vi "Eye Movement Analyser.vi"(7 "Data Output":T12) -> ()   [LabVIEW 2016] (continued)
                  w628 = T14[] [] items=["--- System ---", "Panel Monitoring", "Check Save Status", "Initialize", "Initialise GUI", "Quit", "--- Import ---", "Desaccade Time Data", "Desaccade Time Data Background", "Paint Delete", "Load Batch Log File", "Make Batch List", "Update Batch List", "Delete Batch List", "Delete Temporary LVS", "Save Temporary LVS", "Check for Batch LVS", "Process 3D Chinchilla", "Find default parameter", "Mars3D old", "Chair", "EyeSeeCam", "Open last session", "Save RAW", "Auto Impulse Parameter", "Save Image", "Wireless", "Process Coils Data", "Process JHOC Data", "Process Animal Data", "Australian Data", "ASCII", "Mars 3D", "Mars 3D Training", "Position Mean Plugin", "plot generator plugin", "Human VOG system", "Optotrak", "spline", "COR", "galvanic", "Generate New Time Plot", "Make off and gains permanent", "Generate New Impulse Plot", "Defer Impulse Plot", "Fill Impulse Plot Data", "Scale Impulse Plot", "Un-Defer Impulse Plot", "Snap Impulse Cursor", "Extract Saccades", "Impulse Analyser", "NTA", "Acceleration", "Saccade Velocity", "Horizontal Align", "Vertical Align", "Delete Impulse", "Cut Before", "Cut After", "Filter Data", "Undo Last", "Redo", "Mean and STD", "Group Analyser", "Generate Report", "Phase Plots", "Gain and Phase", "Example Plugin", "Time Constant Plugin", "Export Data", "Export Time Series Data", "Append Data", "Save Data", "Load Data", "Cut in Range", "Keep in range", "Stop"] ("State stack IN")
                  n341 = event-data() -> ()  [unwired: 1 in, 2 out]
                }
                event "Time Constant Plugin": Mouse Down {
                  w631 = T14[] [enum."Time Constant Plugin"] items=["--- System ---", "Panel Monitoring", "Check Save Status", "Initialize", "Initialise GUI", "Quit", "--- Import ---", "Desaccade Time Data", "Desaccade Time Data Background", "Paint Delete", "Load Batch Log File", "Make Batch List", "Update Batch List", "Delete Batch List", "Delete Temporary LVS", "Save Temporary LVS", "Check for Batch LVS", "Process 3D Chinchilla", "Find default parameter", "Mars3D old", "Chair", "EyeSeeCam", "Open last session", "Save RAW", "Auto Impulse Parameter", "Save Image", "Wireless", "Process Coils Data", "Process JHOC Data", "Process Animal Data", "Australian Data", "ASCII", "Mars 3D", "Mars 3D Training", "Position Mean Plugin", "plot generator plugin", "Human VOG system", "Optotrak", "spline", "COR", "galvanic", "Generate New Time Plot", "Make off and gains permanent", "Generate New Impulse Plot", "Defer Impulse Plot", "Fill Impulse Plot Data", "Scale Impulse Plot", "Un-Defer Impulse Plot", "Snap Impulse Cursor", "Extract Saccades", "Impulse Analyser", "NTA", "Acceleration", "Saccade Velocity", "Horizontal Align", "Vertical Align", "Delete Impulse", "Cut Before", "Cut After", "Filter Data", "Undo Last", "Redo", "Mean and STD", "Group Analyser", "Generate Report", "Phase Plots", "Gain and Phase", "Example Plugin", "Time Constant Plugin", "Export Data", "Export Time Series Data", "Append Data", "Save Data", "Load Data", "Cut in Range", "Keep in range", "Stop"] ("State stack IN")
                  n342 = event-data() -> ()  [unwired: 1 in, 8 out]
                }
                event "Main Sequence Saccade": Mouse Down {
                  w634 = T14[] [enum."Extract Saccades"] items=["--- System ---", "Panel Monitoring", "Check Save Status", "Initialize", "Initialise GUI", "Quit", "--- Import ---", "Desaccade Time Data", "Desaccade Time Data Background", "Paint Delete", "Load Batch Log File", "Make Batch List", "Update Batch List", "Delete Batch List", "Delete Temporary LVS", "Save Temporary LVS", "Check for Batch LVS", "Process 3D Chinchilla", "Find default parameter", "Mars3D old", "Chair", "EyeSeeCam", "Open last session", "Save RAW", "Auto Impulse Parameter", "Save Image", "Wireless", "Process Coils Data", "Process JHOC Data", "Process Animal Data", "Australian Data", "ASCII", "Mars 3D", "Mars 3D Training", "Position Mean Plugin", "plot generator plugin", "Human VOG system", "Optotrak", "spline", "COR", "galvanic", "Generate New Time Plot", "Make off and gains permanent", "Generate New Impulse Plot", "Defer Impulse Plot", "Fill Impulse Plot Data", "Scale Impulse Plot", "Un-Defer Impulse Plot", "Snap Impulse Cursor", "Extract Saccades", "Impulse Analyser", "NTA", "Acceleration", "Saccade Velocity", "Horizontal Align", "Vertical Align", "Delete Impulse", "Cut Before", "Cut After", "Filter Data", "Undo Last", "Redo", "Mean and STD", "Group Analyser", "Generate Report", "Phase Plots", "Gain and Phase", "Example Plugin", "Time Constant Plugin", "Export Data", "Export Time Series Data", "Append Data", "Save Data", "Load Data", "Cut in Range", "Keep in range", "Stop"] ("State stack IN")
                  n343 = event-data() -> ()  [unwired: 1 in, 8 out]
                }
                event Menu Selection (User) {
                  n344 = event-data() -> ("ItemTag"=w640:string)  [unwired: 1 in, 6 out]
                  n345 = case shown="\"About\"" w640 {
                    tunnel: [w641 w642 _ w643 w644] -> w637
                    frame "False", Default {
                      w641 = T14[] [enum."Panel Monitoring"] items=["--- System ---", "Panel Monitoring", "Check Save Status", "Initialize", "Initialise GUI", "Quit", "--- Import ---", "Desaccade Time Data", "Desaccade Time Data Background", "Paint Delete", "Load Batch Log File", "Make Batch List", "Update Batch List", "Delete Batch List", "Delete Temporary LVS", "Save Temporary LVS", "Check for Batch LVS", "Process 3D Chinchilla", "Find default parameter", "Mars3D old", "Chair", "EyeSeeCam", "Open last session", "Save RAW", "Auto Impulse Parameter", "Save Image", "Wireless", "Process Coils Data", "Process JHOC Data", "Process Animal Data", "Australian Data", "ASCII", "Mars 3D", "Mars 3D Training", "Position Mean Plugin", "plot generator plugin", "Human VOG system", "Optotrak", "spline", "COR", "galvanic", "Generate New Time Plot", "Make off and gains permanent", "Generate New Impulse Plot", "Defer Impulse Plot", "Fill Impulse Plot Data", "Scale Impulse Plot", "Un-Defer Impulse Plot", "Snap Impulse Cursor", "Extract Saccades", "Impulse Analyser", "NTA", "Acceleration", "Saccade Velocity", "Horizontal Align", "Vertical Align", "Delete Impulse", "Cut Before", "Cut After", "Filter Data", "Undo Last", "Redo", "Mean and STD", "Group Analyser", "Generate Report", "Phase Plots", "Gain and Phase", "Example Plugin", "Time Constant Plugin", "Export Data", "Export Time Series Data", "Append Data", "Save Data", "Load Data", "Cut in Range", "Keep in range", "Stop"]  # State Stack (out)
                    }
                    frame "Load Batch-Log File" {
                      w642 = T14[] [enum."Load Batch Log File"] items=["--- System ---", "Panel Monitoring", "Check Save Status", "Initialize", "Initialise GUI", "Quit", "--- Import ---", "Desaccade Time Data", "Desaccade Time Data Background", "Paint Delete", "Load Batch Log File", "Make Batch List", "Update Batch List", "Delete Batch List", "Delete Temporary LVS", "Save Temporary LVS", "Check for Batch LVS", "Process 3D Chinchilla", "Find default parameter", "Mars3D old", "Chair", "EyeSeeCam", "Open last session", "Save RAW", "Auto Impulse Parameter", "Save Image", "Wireless", "Process Coils Data", "Process JHOC Data", "Process Animal Data", "Australian Data", "ASCII", "Mars 3D", "Mars 3D Training", "Position Mean Plugin", "plot generator plugin", "Human VOG system", "Optotrak", "spline", "COR", "galvanic", "Generate New Time Plot", "Make off and gains permanent", "Generate New Impulse Plot", "Defer Impulse Plot", "Fill Impulse Plot Data", "Scale Impulse Plot", "Un-Defer Impulse Plot", "Snap Impulse Cursor", "Extract Saccades", "Impulse Analyser", "NTA", "Acceleration", "Saccade Velocity", "Horizontal Align", "Vertical Align", "Delete Impulse", "Cut Before", "Cut After", "Filter Data", "Undo Last", "Redo", "Mean and STD", "Group Analyser", "Generate Report", "Phase Plots", "Gain and Phase", "Example Plugin", "Time Constant Plugin", "Export Data", "Export Time Series Data", "Append Data", "Save Data", "Load Data", "Cut in Range", "Keep in range", "Stop"]  # State Stack (out)
                    }
                    frame "About" {
                      n346 = call "About.vi"() -> ()  [unwired: 12 in]
                    }
                    frame "Open" {
                      w643 = T14[] [enum."Load Data"] items=["--- System ---", "Panel Monitoring", "Check Save Status", "Initialize", "Initialise GUI", "Quit", "--- Import ---", "Desaccade Time Data", "Desaccade Time Data Background", "Paint Delete", "Load Batch Log File", "Make Batch List", "Update Batch List", "Delete Batch List", "Delete Temporary LVS", "Save Temporary LVS", "Check for Batch LVS", "Process 3D Chinchilla", "Find default parameter", "Mars3D old", "Chair", "EyeSeeCam", "Open last session", "Save RAW", "Auto Impulse Parameter", "Save Image", "Wireless", "Process Coils Data", "Process JHOC Data", "Process Animal Data", "Australian Data", "ASCII", "Mars 3D", "Mars 3D Training", "Position Mean Plugin", "plot generator plugin", "Human VOG system", "Optotrak", "spline", "COR", "galvanic", "Generate New Time Plot", "Make off and gains permanent", "Generate New Impulse Plot", "Defer Impulse Plot", "Fill Impulse Plot Data", "Scale Impulse Plot", "Un-Defer Impulse Plot", "Snap Impulse Cursor", "Extract Saccades", "Impulse Analyser", "NTA", "Acceleration", "Saccade Velocity", "Horizontal Align", "Vertical Align", "Delete Impulse", "Cut Before", "Cut After", "Filter Data", "Undo Last", "Redo", "Mean and STD", "Group Analyser", "Generate Report", "Phase Plots", "Gain and Phase", "Example Plugin", "Time Constant Plugin", "Export Data", "Export Time Series Data", "Append Data", "Save Data", "Load Data", "Cut in Range", "Keep in range", "Stop"] ("State Stack (out)")
                    }
                    frame "Quit" {
                      w644 = T14[] [enum."Quit"] items=["--- System ---", "Panel Monitoring", "Check Save Status", "Initialize", "Initialise GUI", "Quit", "--- Import ---", "Desaccade Time Data", "Desaccade Time Data Background", "Paint Delete", "Load Batch Log File", "Make Batch List", "Update Batch List", "Delete Batch List", "Delete Temporary LVS", "Save Temporary LVS", "Check for Batch LVS", "Process 3D Chinchilla", "Find default parameter", "Mars3D old", "Chair", "EyeSeeCam", "Open last session", "Save RAW", "Auto Impulse Parameter", "Save Image", "Wireless", "Process Coils Data", "Process JHOC Data", "Process Animal Data", "Australian Data", "ASCII", "Mars 3D", "Mars 3D Training", "Position Mean Plugin", "plot generator plugin", "Human VOG system", "Optotrak", "spline", "COR", "galvanic", "Generate New Time Plot", "Make off and gains permanent", "Generate New Impulse Plot", "Defer Impulse Plot", "Fill Impulse Plot Data", "Scale Impulse Plot", "Un-Defer Impulse Plot", "Snap Impulse Cursor", "Extract Saccades", "Impulse Analyser", "NTA", "Acceleration", "Saccade Velocity", "Horizontal Align", "Vertical Align", "Delete Impulse", "Cut Before", "Cut After", "Filter Data", "Undo Last", "Redo", "Mean and STD", "Group Analyser", "Generate Report", "Phase Plots", "Gain and Phase", "Example Plugin", "Time Constant Plugin", "Export Data", "Export Time Series Data", "Append Data", "Save Data", "Load Data", "Cut in Range", "Keep in range", "Stop"] ("State Stack (out)")
                    }
                  }
                }
                event "Asymmetry Plot": Mouse Up {
                  n347 = event-data() -> ()  [unwired: 1 in, 8 out]
                  n348 = Unbundle By Name(w651) -> ("No. Imp"=w645:i32)
                  n349 = property on="Impulse Trace" class="WFGraph (strict)"() -> ("Value"=w653:cluster{dbl, dbl, "Impulses":dbl[][]})  [unwired: 2 in, 2 out]
                  n350 = Unbundle By Name(w653) -> ("Impulses"=w650:dbl[][])
                  n351 = Array Subset(array=w650, index (row)=0 ("index"), length (row)=w645) -> (w649:dbl[][])  [unwired: 2 in]
                  n352 = Array Subset(array=w650, index (row)=w645) -> (w648:dbl[][])  [unwired: 3 in]
                  n353 = for {
                    tunnel: w649 -> [w656] mode=indexing
                    tunnel: w648 -> [w655] mode=indexing
                    tunnel: [w656] -> w647 mode=concatenating
                    tunnel: [w655] -> w646 mode=concatenating
                  }
                  n354 = call "Asymmetry Plot - Main.vi"("Response"=w646, "Stimulus"=w647) -> ()  [unwired: 10 in]
                }
              }
            }
          }
          n355 = Build Array (concatenate)(w35, w34) -> (w32:T14[])
          n356 = property on="Processing" class="Bool (strict)"("Value"=w29) -> ()  [unwired: 2 in, 2 out]
          n357 = Empty Array?(array=w32) -> (empty?=w33:bool)
        }
      }
      frame "Initialize" {
        w657 = T11 []  # Impulse Positions
        w663 = 100 ("dimension size")
        w669 = TRUE  # Use Excel
        w670 = refnum<k7> refnum  # Excel._Application
        w672 = T14[] [enum."Initialise GUI", enum."Open last session", enum."Make Batch List", enum."Generate New Time Plot", enum."Generate New Impulse Plot", enum."Panel Monitoring"] items=["--- System ---", "Panel Monitoring", "Check Save Status", "Initialize", "Initialise GUI", "Quit", "--- Import ---", "Desaccade Time Data", "Desaccade Time Data Background", "Paint Delete", "Load Batch Log File", "Make Batch List", "Update Batch List", "Delete Batch List", "Delete Temporary LVS", "Save Temporary LVS", "Check for Batch LVS", "Process 3D Chinchilla", "Find default parameter", "Mars3D old", "Chair", "EyeSeeCam", "Open last session", "Save RAW", "Auto Impulse Parameter", "Save Image", "Wireless", "Process Coils Data", "Process JHOC Data", "Process Animal Data", "Australian Data", "ASCII", "Mars 3D", "Mars 3D Training", "Position Mean Plugin", "plot generator plugin", "Human VOG system", "Optotrak", "spline", "COR", "galvanic", "Generate New Time Plot", "Make off and gains permanent", "Generate New Impulse Plot", "Defer Impulse Plot", "Fill Impulse Plot Data", "Scale Impulse Plot", "Un-Defer Impulse Plot", "Snap Impulse Cursor", "Extract Saccades", "Impulse Analyser", "NTA", "Acceleration", "Saccade Velocity", "Horizontal Align", "Vertical Align", "Delete Impulse", "Cut Before", "Cut After", "Filter Data", "Undo Last", "Redo", "Mean and STD", "Group Analyser", "Generate Report", "Phase Plots", "Gain and Phase", "Example Plugin", "Time Constant Plugin", "Export Data", "Export Time Series Data", "Append Data", "Save Data", "Load Data", "Cut in Range", "Keep in range", "Stop"] ("State stack IN")
        w676 = 0  # No. Imp
        # "Important for marking changes to LVS file structure. MUST change if the LVS file structure changes! (See use in Load LVS).\n\n\nIMPORTANT version name MUST be eaxctly 9 characters long."
        # "Mouse Device ID for\nPaint to Delete feature"
        n358 = call <vilib>:"Initialize Mouse.vi"() -> ("device ID"=w666:refnum<k1>)  [unwired: 10 in, 1 out]
        n359 = call "DC_Handler.vi"("Operation"=enum16{"Init", "Set"}."Init") -> ("Event Registration Refnum"=w660:refnum<event-registration>)  [unwired: 10 in]
        n360 = Bundle By Name(cluster=T17 {"Save RAW"=TRUE, "Save Options"=FALSE, "Save IMAGE"=TRUE, "Cycle Nr for Saccades"={"POS"=0, "NEG"=0}, "Paint Delete"=TRUE, "device ID"=refnum, "Delete-Array"=[], "Double Click"=refnum, "DC file"=path "", "Session saved?"=TRUE}, "device ID"=w666, "Double Click"=w660) -> (w667:T17)
        n361 = call "Autosort - Open file.vi"() -> ("Byte Stream File out"=w675:refnum<file>)  [unwired: 11 in]
        n362 = Initialize Array(T18 {"Start"=0, "End"=0, "Impulse Plane"=enum."Other", "Impulse Direction +ve?"=FALSE, "Time offset"=0, "Amplitude offset"=0.0} ("Impulse"), w663, w663) -> (w665:T35)
        n363 = call "Init Statemachine Data TD.vi"() -> ("output cluster"=w674:T30)  [unwired: 2 in]
        n364 = Bundle By Name(cluster=w674, "Old Impulse positions for Undo"=w665, "Impulse Positions"=w657, "No. Imp"=w676, "Autosort File"=w675, "Data File"=T12 {"Data Channels"=[], "Sample Rate"=0, "Channel List"=[]} ("input cluster"), "Histpry Position"=-1) -> (w671:T30)
        n365 = Bundle By Name(cluster=w671, "Excel.Excel._Application"=w670, "Excel.Use Excel"=w669, "EMA Version"="EMA 2016a") -> (w658:T30)
      }
      frame "Initialise GUI" {
        w686 = FALSE ("Visible")
        w690 = TRUE
        w692 = FALSE ("Visible")
        w685 = TRUE ("Visible")
        # "Initialise both graphs to empty"
        n366 = local write "Impulse Plane"(w686) -> ()
        n367 = local write "Saccade Velocity"(w686) -> ()
        n368 = local write "Impulse Parameters"(w686) -> ()
        n369 = property on="Eye Movement Analyser" class="Bool"("Visible"=TRUE) -> ()  [unwired: 2 in, 2 out]
        n370 = property on="Del Autosort" class="Bool (strict)"("Visible"=w685) -> ()  [unwired: 2 in, 2 out]
        n371 = property on="Impulse Characteristics" class="Clust (strict)"("Visible"=w685) -> ()  [unwired: 2 in, 2 out]
        n372 = property on="Impulse Characteristic from Cursor" class="Bool (strict)"("Visible"=w685) -> ()  [unwired: 2 in, 2 out]
        n373 = property on="Autosize Parameter Set" class="Ring (strict)"("Visible"=w685) -> ()  [unwired: 2 in, 2 out]
        n374 = property on="Trigger Channel (Other)" class="Ring (strict)"("Visible"=w685) -> ()  [unwired: 2 in, 2 out]
        n375 = property on="Display Saccade" class="Bool (strict)"("Visible"=w685) -> ()  [unwired: 2 in, 2 out]
        n376 = property on="De-Saccading" class="Bool (strict)"("Val(Sgnl)"=w685) -> ()  [unwired: 2 in, 2 out]
        n377 = property on="Autosize Parameter Set" class="Ring (strict)"("Val(Sgnl)"=i8 0 ("Value (Signaling)")) -> ()  [unwired: 2 in, 2 out]
        n378 = property on="Trigger Method" class="Enum (strict)"("Visible"=w685) -> ()  [unwired: 2 in, 2 out]
        n379 = property on="Default" class="Bool (strict)"("Visible"=w692, "Value"=w692) -> ()  [unwired: 2 in, 2 out]
        n380 = local write "Time series Trace"(cluster{dbl, dbl, dbl[][]} {0.0, 0.005, []} ("Time series Trace")) -> ()
        n381 = local write "Impulse Trace"(cluster{dbl, dbl, "Impulses":dbl[][]} {0.0, 5.0, "Impulses"=[]} ("Impulse Trace")) -> ()
        n382 = local write "calibration filename"("" ("calibration filename")) -> ()
        n383 = property on="Sac Vel" class="Bool"("Visible"=w690) -> ()  [unwired: 2 in, 2 out]
        n384 = property on="Fits a line to a noisy slow-phase. First 3 channels in plot window (above) must be x, y, and z eye position in that order." class="WFGraph (strict)"("Visible"=w690) -> ()  [unwired: 2 in, 2 out]
        n385 = property on="HOR\n\nLARP\n\nRALP" class="Arr (strict)"("Visible"=w690) -> ()  [unwired: 2 in, 2 out]
        n386 = property on="Cross Correlation" class="Bool (strict)"("Visible"=w690) -> ()  [unwired: 2 in, 2 out]
        n387 = property on="Accel Threshold [TH-1]" class="Slide (strict)"("Visible"=w690) -> ()  [unwired: 2 in, 2 out]
        n388 = property on="Tolerance [ms]" class="Slide (strict)"("Visible"=w690) -> ()  [unwired: 2 in, 2 out]
        n389 = property on="X deg/s      Y deg/s      Z deg/s" class="Arr (strict)"("Visible"=w690) -> ()  [unwired: 2 in, 2 out]
        n390 = property on="Add Autosort" class="Bool (strict)"("Visible"=w690) -> ()  [unwired: 2 in, 2 out]
        n391 = property on="Capture Saccade" class="Bool (strict)"("Visible"=w690) -> ()  [unwired: 2 in, 2 out]
        n392 = property on="Impulse surround" class="Clust (strict)"("Visible"=w690) -> ()  [unwired: 2 in, 2 out]
        n393 = local write "Trace"(0 ("Trace")) -> ()
        n394 = property class="App"() -> ("App.Kind"=w680:T36)  [unwired: 2 in, 2 out]
        n395 = property on="Tab Control 3" class="TabCtl (strict)"("Value"=T4."About" ("Tab Control 3")) -> ()  [unwired: 2 in, 2 out]
        n396 = case shown="\"Run Time System\"" w680 {
          frame "invalid app kind", Default {
          }
          frame "Run Time System" {
            w697 = "APP_STOP"  # menu tag
            n397 = Current VI's Menubar() -> (w698:refnum<k9>)
            n398 = Delete Menu Items(8:w697, 9:w698) -> ()  [unwired: 2 in, 2 out]
            n399 = call <userlib>:"Current VIs Reference__ogtk.vi"() -> ("Current VI's reference"=w700:refnum<vi>)  [unwired: 5 in]
            n400 = property class="VI"(reference=w700, "TB.Visible"=FALSE ("Front Panel Window:Custom Title")) -> ()  [unwired: 1 in, 2 out]
          }
          frame "Development System" {
            n401 = call <userlib>:"Current VIs Reference__ogtk.vi"() -> ("Current VI's reference"=w701:refnum<vi>)  [unwired: 5 in]
            n402 = property class="VI"(reference=w701, "TB.Visible"=FALSE ("Front Panel Window:Custom Title")) -> ()  [unwired: 1 in, 2 out]
          }
        }
        n403 = call <userlib>:"Current VIs Reference__ogtk.vi"() -> ("Current VI's reference"=w682:refnum<vi>)  [unwired: 5 in]
        n404 = property class="VI"(reference=w682, "Front Panel.CustomTitle"=TRUE ("Front Panel Window:Custom Title")) -> ()  [unwired: 1 in, 2 out]
      }
      frame "Quit" {
        n405 = Unbundle By Name(w705) -> ("Double Click"=w704:refnum<event-registration>)
        n406 = flat-sequence {
          tunnel: w706 -> [w714]
          frame #0 {
            n407 = Unbundle By Name(w714) -> ("Impulse Positions"=w728:T11, "Old Impulse positions for Undo"=w727:T35, "No. Imp"=w726:i32, "Parameter Time Series"=w725:T2, "Parameter Impuls Series"=w724:T8, "Experiment Parameters"=w723:T25, "Data File"=w722:T12, "Experiment data path"=w721:path, "Image data path"=w720:path, "LVS data path"=w719:path, "Raw copy path"=w718:path, "filename"=w717:string, "desaccading parameters"=w716:T37, "Experiment Parameters 2"=w715:T24, "Autosort Parameter Set"=w711:i32, "calibration name"=w709:string, "Session Config File"=w710:refnum<file>)
            n408 = Bundle("Impulse Positions"=w728, "Old Impulse positions for Undo"=w727, "No. Imp"=w726, "Parameter Time Series"=w725, "Parameter Impuls Series"=w724, "Experiment Parameters"=w723, "Data File"=w722, "Experiment data path"=w721, "Image data path"=w720, "LVS data path"=w719, "Raw copy path"=w718, "filename"=w717, "desaccading parameters"=w716, "Experiment Parameters 2"=w715, "Autosort Parameter Set"=w711, "calibration name"=w709) -> (w712:T38)  [unwired: 1 in]
            n409 = Set File Position(refnum=w710) -> (refnum out=w713:refnum<file>)  [unwired: 3 in, 1 out]
            n410 = Write to Binary File(file (use dialog)=w713, data=w712) -> ()  [unwired: 4 in, 3 out]
          }
          frame #1 {
            n411 = call "Quit LabVIEW if EXE.vi"("Quit LabVIEW?"=TRUE) -> ()  [unwired: 10 in, 1 out]
          }
        }
        n412 = Unregister For Events(event registration refnum=w704) -> ()  [unwired: 1 in, 1 out]
      }
      frame "Stop" {
      }
      frame "--- Import ---" {
      }
      frame "Check for Batch LVS" {
        n413 = property on="Experiment Files" class="MCListbox (strict)"() -> ("ItemNames"=w744:string[][], "Value"=w745:i32)  [unwired: 2 in, 2 out]
        n414 = Unbundle By Name(w752) -> ("Experiment data path"=w741:path)
        n415 = Index Array(array=w744, index (row)=w745, index (col)=0 ("disabled index (col)")) -> (element=w742:string)
        n416 = Build Path(base path=w741, name or relative path=w742) -> (appended path=w740:path)
        n417 = call <vilib>:"Get File Extension.vi"("file"=w740) -> ("filename without extension"=w753:string, "lowercase file extension"=w754:string, "dup file"=w747:path)  [unwired: 6 in, 2 out]
        n418 = disable-structure shown="Enabled" {
          disable-tunnel: w754 -> [w765 w929]
          disable-tunnel: w741 -> [w764 w947]
          disable-tunnel: w753 -> [w763 w944]
          disable-tunnel: w752 -> [w762 w935]
          disable-tunnel: [w761 w934] -> w751
          disable-tunnel: [w760 w930] -> w750
          disable-tunnel: w749 -> [w759 w933]
          disable-tunnel: [w758 w932] -> w748
          disable-tunnel: w747 -> [w757 w931]
          disable-tunnel: w742 -> [w756 _]
          frame Disabled {
            n419 = case shown="\"lvs\"" w765 {
              tunnel: w764 -> [w769 w808 w847 w886 w927]
              tunnel: w763 -> [w778 w817 w856 w895 _]
              tunnel: w762 -> [w772 w811 w850 w889 w925]
              tunnel: [w771 w810 w849 w888 w925] -> w761
              tunnel: [w770 w809 w848 w887 w928] -> w760
              tunnel: w759 -> [w768 w807 w846 w885 w924]
              tunnel: [w767 w806 w845 w884 w923] -> w758
              tunnel: w757 -> [_ _ _ _ w926]
              tunnel: w756 -> [w766 w805 w844 w883 _]
              frame "mars", Default {
                n420 = Concatenate Strings(w778, ".lvs" ("string")) -> (w776:string)
                n421 = Build Path(base path=w769, name or relative path="tmp_batch_lvs") -> (appended path=w780:path)
                n422 = Build Path(base path=w780, name or relative path=w776) -> (appended path=w775:path)
                n423 = call <vilib>:"Check if File or Folder Exists.vi"("path"=w775) -> ("file or folder exists?"=w773:bool, "dup path"=w774:path)  [unwired: 8 in, 1 out]
                n424 = case shown="False" w773 {
                  tunnel: w774 -> [_ w792]
                  tunnel: w772 -> [w786 w794]
                  tunnel: [w786 w793] -> w771
                  tunnel: [w782 w802] -> w770
                  tunnel: w769 -> [w787 w791]
                  tunnel: w768 -> [w785 w801]
                  tunnel: [w784 w801] -> w767
                  tunnel: w766 -> [w781 _]
                  frame False {
                    w782 = T14[] [enum."Mars 3D"] items=["--- System ---", "Panel Monitoring", "Check Save Status", "Initialize", "Initialise GUI", "Quit", "--- Import ---", "Desaccade Time Data", "Desaccade Time Data Background", "Paint Delete", "Load Batch Log File", "Make Batch List", "Update Batch List", "Delete Batch List", "Delete Temporary LVS", "Save Temporary LVS", "Check for Batch LVS", "Process 3D Chinchilla", "Find default parameter", "Mars3D old", "Chair", "EyeSeeCam", "Open last session", "Save RAW", "Auto Impulse Parameter", "Save Image", "Wireless", "Process Coils Data", "Process JHOC Data", "Process Animal Data", "Australian Data", "ASCII", "Mars 3D", "Mars 3D Training", "Position Mean Plugin", "plot generator plugin", "Human VOG system", "Optotrak", "spline", "COR", "galvanic", "Generate New Time Plot", "Make off and gains permanent", "Generate New Impulse Plot", "Defer Impulse Plot", "Fill Impulse Plot Data", "Scale Impulse Plot", "Un-Defer Impulse Plot", "Snap Impulse Cursor", "Extract Saccades", "Impulse Analyser", "NTA", "Acceleration", "Saccade Velocity", "Horizontal Align", "Vertical Align", "Delete Impulse", "Cut Before", "Cut After", "Filter Data", "Undo Last", "Redo", "Mean and STD", "Group Analyser", "Generate Report", "Phase Plots", "Gain and Phase", "Example Plugin", "Time Constant Plugin", "Export Data", "Export Time Series Data", "Append Data", "Save Data", "Load Data", "Cut in Range", "Keep in range", "Stop"] ("State stack OUT")
                    n425 = Build Path(base path=w787, name or relative path=w781) -> (appended path=w783:path)
                    n426 = Bundle By Name(cluster=w785, "DC file"=w783) -> (w784:T17)
                  }
                  frame True {
                    w802 = T14[] [enum."Panel Monitoring", enum."Generate New Time Plot", enum."Generate New Impulse Plot"] items=["--- System ---", "Panel Monitoring", "Check Save Status", "Initialize", "Initialise GUI", "Quit", "--- Import ---", "Desaccade Time Data", "Desaccade Time Data Background", "Paint Delete", "Load Batch Log File", "Make Batch List", "Update Batch List", "Delete Batch List", "Delete Temporary LVS", "Save Temporary LVS", "Check for Batch LVS", "Process 3D Chinchilla", "Find default parameter", "Mars3D old", "Chair", "EyeSeeCam", "Open last session", "Save RAW", "Auto Impulse Parameter", "Save Image", "Wireless", "Process Coils Data", "Process JHOC Data", "Process Animal Data", "Australian Data", "ASCII", "Mars 3D", "Mars 3D Training", "Position Mean Plugin", "plot generator plugin", "Human VOG system", "Optotrak", "spline", "COR", "galvanic", "Generate New Time Plot", "Make off and gains permanent", "Generate New Impulse Plot", "Defer Impulse Plot", "Fill Impulse Plot Data", "Scale Impulse Plot", "Un-Defer Impulse Plot", "Snap Impulse Cursor", "Extract Saccades", "Impulse Analyser", "NTA", "Acceleration", "Saccade Velocity", "Horizontal Align", "Vertical Align", "Delete Impulse", "Cut Before", "Cut After", "Filter Data", "Undo Last", "Redo", "Mean and STD", "Group Analyser", "Generate Report", "Phase Plots", "Gain and Phase", "Example Plugin", "Time Constant Plugin", "Export Data", "Export Time Series Data", "Append Data", "Save Data", "Load Data", "Cut in Range", "Keep in range", "Stop"] ("State stack OUT")
                    n427 = call <vilib>:"Open_Create_Replace File.vi"("function (open:0)"=T19."open", "file path"=w792) -> ("refnum"=w804:refnum<file>)  [unwired: 6 in, 3 out]
                    n428 = property on="Experiment Files" class="MCListbox (strict)"() -> ("ItemNames"=w799:string[][], "Value"=w798:i32)  [unwired: 2 in, 2 out]
                    n429 = call <vilib>:"Read File+ (string).vi"("count"=9, "refnum"=w804) -> ("dup refnum"=w789:refnum<file>)  [unwired: 5 in, 4 out]
                    n430 = Replace Array Subset(array=w799, new element="LVS" ("new element/subarray"), index (row)=w798, index (col)=1 ("disabled index (col)")) -> (w795:string[][])
                    n431 = call "Update Batch XML.vi"("ItemNames"=w795, "Data OUT"=w794) -> ()  [unwired: 10 in]
                    n432 = property on="Experiment Files" class="MCListbox (strict)"("ItemNames"=w795) -> ()  [unwired: 2 in, 2 out]
                    n433 = call "Load LVS EMA 2010b.vi"("Data OUT in"=w794, "Byte Stream File in"=w789) -> ("Byte Stream File out"=w788:refnum<file>, "Data OUT out"=w790:T30)  [unwired: 8 in]
                    n434 = Bundle By Name(cluster=w790, "Experiment data path"=w791) -> (w793:T30)
                    n435 = Close File(refnum=w788) -> ()  [unwired: 1 in, 2 out]
                  }
                }
              }
              frame "hrch" {
                n436 = Concatenate Strings(w817, ".lvs" ("string")) -> (w815:string)
                n437 = Build Path(base path=w808, name or relative path="tmp_batch_lvs") -> (appended path=w819:path)
                n438 = Build Path(base path=w819, name or relative path=w815) -> (appended path=w814:path)
                n439 = call <vilib>:"Check if File or Folder Exists.vi"("path"=w814) -> ("file or folder exists?"=w812:bool, "dup path"=w813:path)  [unwired: 8 in, 1 out]
                n440 = case shown="False" w812 {
                  tunnel: w813 -> [_ w830]
                  tunnel: w811 -> [w825 w832]
                  tunnel: [w825 w831] -> w810
                  tunnel: [w821 w840] -> w809
                  tunnel: w808 -> [w826 w829]
                  tunnel: w807 -> [w824 w839]
                  tunnel: [w823 w839] -> w806
                  tunnel: w805 -> [w820 _]
                  frame False {
                    w821 = T14[] [enum."Chair"] items=["--- System ---", "Panel Monitoring", "Check Save Status", "Initialize", "Initialise GUI", "Quit", "--- Import ---", "Desaccade Time Data", "Desaccade Time Data Background", "Paint Delete", "Load Batch Log File", "Make Batch List", "Update Batch List", "Delete Batch List", "Delete Temporary LVS", "Save Temporary LVS", "Check for Batch LVS", "Process 3D Chinchilla", "Find default parameter", "Mars3D old", "Chair", "EyeSeeCam", "Open last session", "Save RAW", "Auto Impulse Parameter", "Save Image", "Wireless", "Process Coils Data", "Process JHOC Data", "Process Animal Data", "Australian Data", "ASCII", "Mars 3D", "Mars 3D Training", "Position Mean Plugin", "plot generator plugin", "Human VOG system", "Optotrak", "spline", "COR", "galvanic", "Generate New Time Plot", "Make off and gains permanent", "Generate New Impulse Plot", "Defer Impulse Plot", "Fill Impulse Plot Data", "Scale Impulse Plot", "Un-Defer Impulse Plot", "Snap Impulse Cursor", "Extract Saccades", "Impulse Analyser", "NTA", "Acceleration", "Saccade Velocity", "Horizontal Align", "Vertical Align", "Delete Impulse", "Cut Before", "Cut After", "Filter Data", "Undo Last", "Redo", "Mean and STD", "Group Analyser", "Generate Report", "Phase Plots", "Gain and Phase", "Example Plugin", "Time Constant Plugin", "Export Data", "Export Time Series Data", "Append Data", "Save Data", "Load Data", "Cut in Range", "Keep in range", "Stop"] ("State stack OUT")
                    n441 = Build Path(base path=w826, name or relative path=w820) -> (appended path=w822:path)
                    n442 = Bundle By Name(cluster=w824, "DC file"=w822) -> (w823:T17)
                  }
                  frame True {
                    w840 = T14[] [enum."Panel Monitoring", enum."Generate New Time Plot", enum."Generate New Impulse Plot"] items=["--- System ---", "Panel Monitoring", "Check Save Status", "Initialize", "Initialise GUI", "Quit", "--- Import ---", "Desaccade Time Data", "Desaccade Time Data Background", "Paint Delete", "Load Batch Log File", "Make Batch List", "Update Batch List", "Delete Batch List", "Delete Temporary LVS", "Save Temporary LVS", "Check for Batch LVS", "Process 3D Chinchilla", "Find default parameter", "Mars3D old", "Chair", "EyeSeeCam", "Open last session", "Save RAW", "Auto Impulse Parameter", "Save Image", "Wireless", "Process Coils Data", "Process JHOC Data", "Process Animal Data", "Australian Data", "ASCII", "Mars 3D", "Mars 3D Training", "Position Mean Plugin", "plot generator plugin", "Human VOG system", "Optotrak", "spline", "COR", "galvanic", "Generate New Time Plot", "Make off and gains permanent", "Generate New Impulse Plot", "Defer Impulse Plot", "Fill Impulse Plot Data", "Scale Impulse Plot", "Un-Defer Impulse Plot", "Snap Impulse Cursor", "Extract Saccades", "Impulse Analyser", "NTA", "Acceleration", "Saccade Velocity", "Horizontal Align", "Vertical Align", "Delete Impulse", "Cut Before", "Cut After", "Filter Data", "Undo Last", "Redo", "Mean and STD", "Group Analyser", "Generate Report", "Phase Plots", "Gain and Phase", "Example Plugin", "Time Constant Plugin", "Export Data", "Export Time Series Data", "Append Data", "Save Data", "Load Data", "Cut in Range", "Keep in range", "Stop"] ("State stack OUT")
                    n443 = call <vilib>:"Open_Create_Replace File.vi"("function (open:0)"=T19."open", "file path"=w830) -> ("refnum"=w843:refnum<file>)  [unwired: 6 in, 3 out]
                    n444 = call <vilib>:"Read File+ (string).vi"("count"=9, "refnum"=w843) -> ("dup refnum"=w841:refnum<file>)  [unwired: 5 in, 4 out]
                    n445 = property on="Experiment Files" class="MCListbox (strict)"() -> ("ItemNames"=w837:string[][], "Value"=w836:i32)  [unwired: 2 in, 2 out]
                    n446 = Replace Array Subset(array=w837, new element="LVS" ("new element/subarray"), index (row)=w836, index (col)=1 ("disabled index (col)")) -> (w833:string[][])
                    n447 = call "Load LVS EMA 2010b.vi"("Data OUT in"=w832, "Byte Stream File in"=w841) -> ("Byte Stream File out"=w827:refnum<file>, "Data OUT out"=w828:T30)  [unwired: 8 in]
                    n448 = property on="Experiment Files" class="MCListbox (strict)"("ItemNames"=w833) -> ()  [unwired: 2 in, 2 out]
                    n449 = call "Update Batch XML.vi"("ItemNames"=w833, "Data OUT"=w832) -> ()  [unwired: 10 in]
                    n450 = Bundle By Name(cluster=w828, "Experiment data path"=w829) -> (w831:T30)
                    n451 = Close File(refnum=w827) -> ()  [unwired: 1 in, 2 out]
                  }
                }
              }
              frame "mat" {
                n452 = Concatenate Strings(w856, ".lvs" ("string")) -> (w854:string)
                n453 = Build Path(base path=w847, name or relative path="tmp_batch_lvs") -> (appended path=w858:path)
                n454 = Build Path(base path=w858, name or relative path=w854) -> (appended path=w853:path)
                n455 = call <vilib>:"Check if File or Folder Exists.vi"("path"=w853) -> ("file or folder exists?"=w851:bool, "dup path"=w852:path)  [unwired: 8 in, 1 out]
                n456 = case shown="False" w851 {
                  tunnel: w852 -> [_ w874]
                  tunnel: w850 -> [w864 w876]
                  tunnel: [w864 w875] -> w849
                  tunnel: [w860 w879] -> w848
                  tunnel: w847 -> [w865 w873]
                  tunnel: w846 -> [w863 w878]
                  tunnel: [w862 w878] -> w845
                  tunnel: w844 -> [w859 _]
                  frame False {
                    w860 = T14[] [enum."EyeSeeCam"] items=["--- System ---", "Panel Monitoring", "Check Save Status", "Initialize", "Initialise GUI", "Quit", "--- Import ---", "Desaccade Time Data", "Desaccade Time Data Background", "Paint Delete", "Load Batch Log File", "Make Batch List", "Update Batch List", "Delete Batch List", "Delete Temporary LVS", "Save Temporary LVS", "Check for Batch LVS", "Process 3D Chinchilla", "Find default parameter", "Mars3D old", "Chair", "EyeSeeCam", "Open last session", "Save RAW", "Auto Impulse Parameter", "Save Image", "Wireless", "Process Coils Data", "Process JHOC Data", "Process Animal Data", "Australian Data", "ASCII", "Mars 3D", "Mars 3D Training", "Position Mean Plugin", "plot generator plugin", "Human VOG system", "Optotrak", "spline", "COR", "galvanic", "Generate New Time Plot", "Make off and gains permanent", "Generate New Impulse Plot", "Defer Impulse Plot", "Fill Impulse Plot Data", "Scale Impulse Plot", "Un-Defer Impulse Plot", "Snap Impulse Cursor", "Extract Saccades", "Impulse Analyser", "NTA", "Acceleration", "Saccade Velocity", "Horizontal Align", "Vertical Align", "Delete Impulse", "Cut Before", "Cut After", "Filter Data", "Undo Last", "Redo", "Mean and STD", "Group Analyser", "Generate Report", "Phase Plots", "Gain and Phase", "Example Plugin", "Time Constant Plugin", "Export Data", "Export Time Series Data", "Append Data", "Save Data", "Load Data", "Cut in Range", "Keep in range", "Stop"] ("State stack OUT")
                    n457 = Build Path(base path=w865, name or relative path=w859) -> (appended path=w861:path)
                    n458 = Bundle By Name(cluster=w863, "DC file"=w861) -> (w862:T17)
                  }
                  frame True {
                    w879 = T14[] [enum."Panel Monitoring", enum."Generate New Time Plot", enum."Generate New Impulse Plot"] items=["--- System ---", "Panel Monitoring", "Check Save Status", "Initialize", "Initialise GUI", "Quit", "--- Import ---", "Desaccade Time Data", "Desaccade Time Data Background", "Paint Delete", "Load Batch Log File", "Make Batch List", "Update Batch List", "Delete Batch List", "Delete Temporary LVS", "Save Temporary LVS", "Check for Batch LVS", "Process 3D Chinchilla", "Find default parameter", "Mars3D old", "Chair", "EyeSeeCam", "Open last session", "Save RAW", "Auto Impulse Parameter", "Save Image", "Wireless", "Process Coils Data", "Process JHOC Data", "Process Animal Data", "Australian Data", "ASCII", "Mars 3D", "Mars 3D Training", "Position Mean Plugin", "plot generator plugin", "Human VOG system", "Optotrak", "spline", "COR", "galvanic", "Generate New Time Plot", "Make off and gains permanent", "Generate New Impulse Plot", "Defer Impulse Plot", "Fill Impulse Plot Data", "Scale Impulse Plot", "Un-Defer Impulse Plot", "Snap Impulse Cursor", "Extract Saccades", "Impulse Analyser", "NTA", "Acceleration", "Saccade Velocity", "Horizontal Align", "Vertical Align", "Delete Impulse", "Cut Before", "Cut After", "Filter Data", "Undo Last", "Redo", "Mean and STD", "Group Analyser", "Generate Report", "Phase Plots", "Gain and Phase", "Example Plugin", "Time Constant Plugin", "Export Data", "Export Time Series Data", "Append Data", "Save Data", "Load Data", "Cut in Range", "Keep in range", "Stop"] ("State stack OUT")
                    n459 = call <vilib>:"Open_Create_Replace File.vi"("function (open:0)"=T19."open", "file path"=w874) -> ("refnum"=w882:refnum<file>)  [unwired: 6 in, 3 out]
                    n460 = call <vilib>:"Read File+ (string).vi"("count"=9, "refnum"=w882) -> ("dup refnum"=w880:refnum<file>)  [unwired: 5 in, 4 out]
                    n461 = property on="Experiment Files" class="MCListbox (strict)"() -> ("ItemNames"=w870:string[][], "Value"=w869:i32)  [unwired: 2 in, 2 out]
                    n462 = Replace Array Subset(array=w870, new element="LVS" ("new element/subarray"), index (row)=w869, index (col)=1 ("disabled index (col)")) -> (w866:string[][])
                    n463 = call "Load LVS EMA 2010b.vi"("Data OUT in"=w876, "Byte Stream File in"=w880) -> ("Byte Stream File out"=w871:refnum<file>, "Data OUT out"=w872:T30)  [unwired: 8 in]
                    n464 = property on="Experiment Files" class="MCListbox (strict)"("ItemNames"=w866) -> ()  [unwired: 2 in, 2 out]
                    n465 = call "Update Batch XML.vi"("ItemNames"=w866, "Data OUT"=w876) -> ()  [unwired: 10 in]
                    n466 = Bundle By Name(cluster=w872, "Experiment data path"=w873) -> (w875:T30)
                    n467 = Close File(refnum=w871) -> ()  [unwired: 1 in, 2 out]
                  }
                }
              }
              frame "raw" {
                n468 = Concatenate Strings(w895, ".lvs" ("string")) -> (w893:string)
                n469 = Build Path(base path=w886, name or relative path="tmp_batch_lvs") -> (appended path=w897:path)
                n470 = Build Path(base path=w897, name or relative path=w893) -> (appended path=w892:path)
                n471 = call <vilib>:"Check if File or Folder Exists.vi"("path"=w892) -> ("file or folder exists?"=w890:bool, "dup path"=w891:path)  [unwired: 8 in, 1 out]
                n472 = case shown="False" w890 {
                  tunnel: w891 -> [_ w909]
                  tunnel: w889 -> [w903 w911]
                  tunnel: [w903 w910] -> w888
                  tunnel: [w899 w919] -> w887
                  tunnel: w886 -> [w904 w908]
                  tunnel: w885 -> [w902 w918]
                  tunnel: [w901 w918] -> w884
                  tunnel: w883 -> [w898 _]
                  frame False {
                    w899 = T14[] [enum."Process JHOC Data"] items=["--- System ---", "Panel Monitoring", "Check Save Status", "Initialize", "Initialise GUI", "Quit", "--- Import ---", "Desaccade Time Data", "Desaccade Time Data Background", "Paint Delete", "Load Batch Log File", "Make Batch List", "Update Batch List", "Delete Batch List", "Delete Temporary LVS", "Save Temporary LVS", "Check for Batch LVS", "Process 3D Chinchilla", "Find default parameter", "Mars3D old", "Chair", "EyeSeeCam", "Open last session", "Save RAW", "Auto Impulse Parameter", "Save Image", "Wireless", "Process Coils Data", "Process JHOC Data", "Process Animal Data", "Australian Data", "ASCII", "Mars 3D", "Mars 3D Training", "Position Mean Plugin", "plot generator plugin", "Human VOG system", "Optotrak", "spline", "COR", "galvanic", "Generate New Time Plot", "Make off and gains permanent", "Generate New Impulse Plot", "Defer Impulse Plot", "Fill Impulse Plot Data", "Scale Impulse Plot", "Un-Defer Impulse Plot", "Snap Impulse Cursor", "Extract Saccades", "Impulse Analyser", "NTA", "Acceleration", "Saccade Velocity", "Horizontal Align", "Vertical Align", "Delete Impulse", "Cut Before", "Cut After", "Filter Data", "Undo Last", "Redo", "Mean and STD", "Group Analyser", "Generate Report", "Phase Plots", "Gain and Phase", "Example Plugin", "Time Constant Plugin", "Export Data", "Export Time Series Data", "Append Data", "Save Data", "Load Data", "Cut in Range", "Keep in range", "Stop"] ("State stack OUT")
                    n473 = Build Path(base path=w904, name or relative path=w898) -> (appended path=w900:path)
                    n474 = Bundle By Name(cluster=w902, "DC file"=w900) -> (w901:T17)
                  }
                  frame True {
                    w919 = T14[] [enum."Panel Monitoring", enum."Generate New Time Plot", enum."Generate New Impulse Plot"] items=["--- System ---", "Panel Monitoring", "Check Save Status", "Initialize", "Initialise GUI", "Quit", "--- Import ---", "Desaccade Time Data", "Desaccade Time Data Background", "Paint Delete", "Load Batch Log File", "Make Batch List", "Update Batch List", "Delete Batch List", "Delete Temporary LVS", "Save Temporary LVS", "Check for Batch LVS", "Process 3D Chinchilla", "Find default parameter", "Mars3D old", "Chair", "EyeSeeCam", "Open last session", "Save RAW", "Auto Impulse Parameter", "Save Image", "Wireless", "Process Coils Data", "Process JHOC Data", "Process Animal Data", "Australian Data", "ASCII", "Mars 3D", "Mars 3D Training", "Position Mean Plugin", "plot generator plugin", "Human VOG system", "Optotrak", "spline", "COR", "galvanic", "Generate New Time Plot", "Make off and gains permanent", "Generate New Impulse Plot", "Defer Impulse Plot", "Fill Impulse Plot Data", "Scale Impulse Plot", "Un-Defer Impulse Plot", "Snap Impulse Cursor", "Extract Saccades", "Impulse Analyser", "NTA", "Acceleration", "Saccade Velocity", "Horizontal Align", "Vertical Align", "Delete Impulse", "Cut Before", "Cut After", "Filter Data", "Undo Last", "Redo", "Mean and STD", "Group Analyser", "Generate Report", "Phase Plots", "Gain and Phase", "Example Plugin", "Time Constant Plugin", "Export Data", "Export Time Series Data", "Append Data", "Save Data", "Load Data", "Cut in Range", "Keep in range", "Stop"] ("State stack OUT")
                    n475 = property on="Experiment Files" class="MCListbox (strict)"() -> ("ItemNames"=w916:string[][], "Value"=w915:i32)  [unwired: 2 in, 2 out]
                    n476 = call <vilib>:"Open_Create_Replace File.vi"("function (open:0)"=T19."open", "file path"=w909) -> ("refnum"=w921:refnum<file>)  [unwired: 6 in, 3 out]
                    n477 = call <vilib>:"Read File+ (string).vi"("count"=9, "refnum"=w921) -> ("dup refnum"=w906:refnum<file>)  [unwired: 5 in, 4 out]
                    n478 = Replace Array Subset(array=w916, new element="LVS" ("new element/subarray"), index (row)=w915, index (col)=1 ("disabled index (col)")) -> (w912:string[][])
                    n479 = property on="Experiment Files" class="MCListbox (strict)"("ItemNames"=w912) -> ()  [unwired: 2 in, 2 out]
                    n480 = call "Update Batch XML.vi"("ItemNames"=w912, "Data OUT"=w911) -> ()  [unwired: 10 in]
                    n481 = call "Load LVS EMA 2010b.vi"("Data OUT in"=w911, "Byte Stream File in"=w906) -> ("Byte Stream File out"=w905:refnum<file>, "Data OUT out"=w907:T30)  [unwired: 8 in]
                    n482 = Close File(refnum=w905) -> ()  [unwired: 1 in, 2 out]
                    n483 = Bundle By Name(cluster=w907, "Experiment data path"=w908) -> (w910:T30)
                  }
                }
              }
              frame "lvs" {
                w928 = T14[] [enum."Load Data", enum."Generate New Time Plot", enum."Generate New Impulse Plot"] items=["--- System ---", "Panel Monitoring", "Check Save Status", "Initialize", "Initialise GUI", "Quit", "--- Import ---", "Desaccade Time Data", "Desaccade Time Data Background", "Paint Delete", "Load Batch Log File", "Make Batch List", "Update Batch List", "Delete Batch List", "Delete Temporary LVS", "Save Temporary LVS", "Check for Batch LVS", "Process 3D Chinchilla", "Find default parameter", "Mars3D old", "Chair", "EyeSeeCam", "Open last session", "Save RAW", "Auto Impulse Parameter", "Save Image", "Wireless", "Process Coils Data", "Process JHOC Data", "Process Animal Data", "Australian Data", "ASCII", "Mars 3D", "Mars 3D Training", "Position Mean Plugin", "plot generator plugin", "Human VOG system", "Optotrak", "spline", "COR", "galvanic", "Generate New Time Plot", "Make off and gains permanent", "Generate New Impulse Plot", "Defer Impulse Plot", "Fill Impulse Plot Data", "Scale Impulse Plot", "Un-Defer Impulse Plot", "Snap Impulse Cursor", "Extract Saccades", "Impulse Analyser", "NTA", "Acceleration", "Saccade Velocity", "Horizontal Align", "Vertical Align", "Delete Impulse", "Cut Before", "Cut After", "Filter Data", "Undo Last", "Redo", "Mean and STD", "Group Analyser", "Generate Report", "Phase Plots", "Gain and Phase", "Example Plugin", "Time Constant Plugin", "Export Data", "Export Time Series Data", "Append Data", "Save Data", "Load Data", "Cut in Range", "Keep in range", "Stop"] ("State stack OUT")
                n484 = Build Path(base path=w927, name or relative path=w926) -> (appended path=w922:path)
                n485 = Bundle By Name(cluster=w924, "DC file"=w922) -> (w923:T17)
              }
            }
          }
          frame Enabled {
            n486 = Build Path(base path=w947, name or relative path="tmp_batch_lvs") -> (appended path=w942:path)
            n487 = Concatenate Strings(w944, ".lvs" ("string")) -> (w941:string)
            n488 = Equal?(x=w929, y="lvs" ("string")) -> (x = y?=w936:bool)
            n489 = Build Path(base path=w942, name or relative path=w941) -> (appended path=w943:path)
            n490 = call <vilib>:"Check if File or Folder Exists.vi"("path"=w943) -> ("file or folder exists?"=w937:bool, "dup path"=w938:path)  [unwired: 8 in, 1 out]
            n491 = Or(x=w937, y=w936) -> (x .or. y?=w939:bool)
            n492 = case shown="True" w939 {
              tunnel: w938 -> [_ w968]
              tunnel: w936 -> [_ w969]
              tunnel: w935 -> [w949 w967]
              tunnel: [w949 w967] -> w934
              tunnel: w933 -> [w952 w966]
              tunnel: [w951 w965] -> w932
              tunnel: w931 -> [w950 w964]
              tunnel: [w948 w962] -> w930
              tunnel: w929 -> [w953 _]
              frame False {
                # "This is the file that will be loaded by the Load Data State."
                # "Some other file type was selected. Load it."
                n493 = case shown="\"raw\"" w953 {
                  selector: w953 -> [w956 _ _ _ _]
                  tunnel: [w954 w958 w959 w960 w961] -> w948
                  frame Default {
                    w954 = T14[] [enum."Panel Monitoring"] items=["--- System ---", "Panel Monitoring", "Check Save Status", "Initialize", "Initialise GUI", "Quit", "--- Import ---", "Desaccade Time Data", "Desaccade Time Data Background", "Paint Delete", "Load Batch Log File", "Make Batch List", "Update Batch List", "Delete Batch List", "Delete Temporary LVS", "Save Temporary LVS", "Check for Batch LVS", "Process 3D Chinchilla", "Find default parameter", "Mars3D old", "Chair", "EyeSeeCam", "Open last session", "Save RAW", "Auto Impulse Parameter", "Save Image", "Wireless", "Process Coils Data", "Process JHOC Data", "Process Animal Data", "Australian Data", "ASCII", "Mars 3D", "Mars 3D Training", "Position Mean Plugin", "plot generator plugin", "Human VOG system", "Optotrak", "spline", "COR", "galvanic", "Generate New Time Plot", "Make off and gains permanent", "Generate New Impulse Plot", "Defer Impulse Plot", "Fill Impulse Plot Data", "Scale Impulse Plot", "Un-Defer Impulse Plot", "Snap Impulse Cursor", "Extract Saccades", "Impulse Analyser", "NTA", "Acceleration", "Saccade Velocity", "Horizontal Align", "Vertical Align", "Delete Impulse", "Cut Before", "Cut After", "Filter Data", "Undo Last", "Redo", "Mean and STD", "Group Analyser", "Generate Report", "Phase Plots", "Gain and Phase", "Example Plugin", "Time Constant Plugin", "Export Data", "Export Time Series Data", "Append Data", "Save Data", "Load Data", "Cut in Range", "Keep in range", "Stop"] ("State stack OUT")
                    # "Unknown. Throw Error Message."
                    n494 = Concatenate Strings("Unknown file type: ", w956) -> (w955:string)
                    n495 = One Button Dialog(message=w955) -> ()  [unwired: 1 in, 1 out]
                  }
                  frame "hrch" {
                    w958 = T14[] [enum."Chair"] items=["--- System ---", "Panel Monitoring", "Check Save Status", "Initialize", "Initialise GUI", "Quit", "--- Import ---", "Desaccade Time Data", "Desaccade Time Data Background", "Paint Delete", "Load Batch Log File", "Make Batch List", "Update Batch List", "Delete Batch List", "Delete Temporary LVS", "Save Temporary LVS", "Check for Batch LVS", "Process 3D Chinchilla", "Find default parameter", "Mars3D old", "Chair", "EyeSeeCam", "Open last session", "Save RAW", "Auto Impulse Parameter", "Save Image", "Wireless", "Process Coils Data", "Process JHOC Data", "Process Animal Data", "Australian Data", "ASCII", "Mars 3D", "Mars 3D Training", "Position Mean Plugin", "plot generator plugin", "Human VOG system", "Optotrak", "spline", "COR", "galvanic", "Generate New Time Plot", "Make off and gains permanent", "Generate New Impulse Plot", "Defer Impulse Plot", "Fill Impulse Plot Data", "Scale Impulse Plot", "Un-Defer Impulse Plot", "Snap Impulse Cursor", "Extract Saccades", "Impulse Analyser", "NTA", "Acceleration", "Saccade Velocity", "Horizontal Align", "Vertical Align", "Delete Impulse", "Cut Before", "Cut After", "Filter Data", "Undo Last", "Redo", "Mean and STD", "Group Analyser", "Generate Report", "Phase Plots", "Gain and Phase", "Example Plugin", "Time Constant Plugin", "Export Data", "Export Time Series Data", "Append Data", "Save Data", "Load Data", "Cut in Range", "Keep in range", "Stop"] ("State stack OUT")
                    # "Human Rotary Chair"
                  }
                  frame "mat" {
